vi "SD-Typecast Queue to Refnum.vi"(11 "queue in":T1) -> (3 "refnum out":T2)   [LabVIEW 2020, in "SD-NI_LVConfig.lvlib"]
uses:
  SD-NI_LVConfig.lvlib
  SD-Config Data RefNum.ctl
  SD-Section.ctl
  <vilib>/Utility/config.llb/Config Data.ctl
  <vilib>/Utility/config.llb/Config Queue.ctl
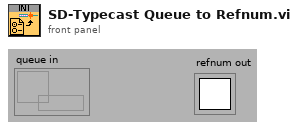
[diagram p1: front panel]
types:
  T1 = typedef "NI_LVConfig.lvlib/Config Queue.ctl" = refnum<queue>
  T2 = typedef "SD-NI_LVConfig.lvlib/SD-Config Data RefNum.ctl" = refnum<k1>
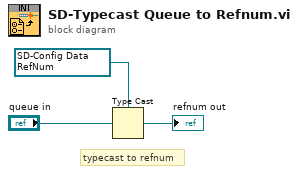
[diagram p0: block diagram]
diagram:
  w2 = T2 refnum items=["config data"] ("refnum out")
  # "typecast to refnum"
  n1 = Type Cast(type=w2, x="queue in") -> (*(type *) &x=→"refnum out":T2)
